vi "Untitled 3.vi"() -> ()   [LabVIEW 2014]
uses:
  <vilib>/Instr/_visa.llb/VISA Configure Serial Port (Instr).vi
panel:
  out "y-position":dbl
  out "z-position":dbl
  out "x-position":dbl
  out "read buffer":string
  in  "write buffer":string
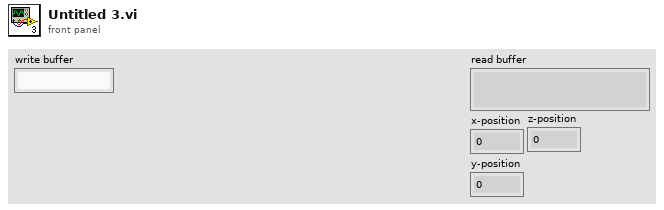
[diagram p1: front panel]
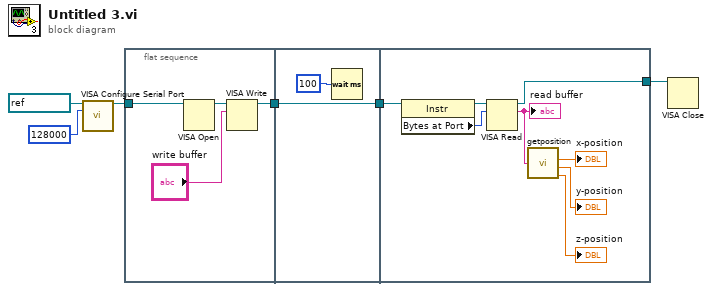
[diagram p0: block diagram]
diagram:
  n1 = call-poly "VISA Configure Serial Port"("VISA resource name"=refnum<visa-resource-name> "COM2", "baud rate (9600)"=u32 128000) -> ("VISA resource name out"=w4:refnum<visa-resource-name>)  [unwired: 12 in, 1 out]
  n2 = flat-sequence {
    tunnel: w4 -> [w10]
    tunnel: [w7] -> w2
    tunnel: [w11] -> w3
    tunnel: w2 -> [w11]
    tunnel: w3 -> [w19]
    tunnel: [w17] -> w1
    frame #0 {
      n3 = VISA Open(VISA resource name=w10) -> (VISA resource name=w9:refnum<visa-resource-name>)  [unwired: 4 in, 1 out]
      n4 = VISA Write(VISA resource name=w9, write buffer="write buffer") -> (VISA resource name out=w7:refnum<visa-resource-name>)  [unwired: 1 in, 2 out]
    }
    frame #1 {
      n5 = Wait (ms)(milliseconds to wait=u32 100) -> ()  [unwired: 1 out]
    }
    frame #2 {
      n6 = property class="Instr"(reference=w19) -> (reference out=w20:refnum<visa-resource-name>, "Bytes at Port"=w18:u32)  [unwired: 1 in, 1 out]
      n7 = VISA Read(VISA resource name=w20, byte count=w18) -> (VISA resource name out=w17:refnum<visa-resource-name>, read buffer=w16:string)  [unwired: 1 in, 2 out]
      "read buffer" <- w16
      n8 = call "getposition.vi"("string"=w16) -> ("x-position"=→"x-position":dbl, "y-position"=→"y-position":dbl, "z-position"=→"z-position":dbl)  [unwired: 1 out]
    }
  }
  n9 = VISA Close(VISA resource name=w1) -> ()  [unwired: 1 in, 1 out]
